vi "DylanScreenTest.vi"() -> ()   [LabVIEW 2019]
uses:
  <userlib>/MicroPython/VIs/uPythonX/uPythonX.xctl
panel:
  in  "Examples":T1(xcontrol)={"VISA Refnum in"="ASRL44::INSTR", "Python Code"="# MicroPython SSD1327 OLED driver examples\n\n# WeMos D1 Mini -- Grove OLED 96x96\n# D1 GPIO5 ------- SCL\n# D2 GPIO4 ------- SDA\n# 3V3 ------------ VCC\n# GND ------------ GND\n\nimport ssd1327\nfrom machine import I2C, Pin\n\n# generic 128x128 SSD1327 OLED\n# i2c = I2C(sda=Pin(4), scl=Pin(5))\n# display = ssd1327.SSD1327_I2C(96, 96, i2c, 60)\n\n# Seeed 96x96 SSD1327 OLED\n#i2c = I2C(sda=Pin(4), scl=Pin(5))\ni2c = I2C(2)\ndisplay = ssd1327.SEEED_OLED_96X96(i2c)\n\n\n# hello world\nfor y in range(0,12):\n     display.text('Hello World', 0, y * 8, 15 - y)\ndisplay.show()\n\n\n# 15 shades of grey\ndisplay.fill(0)\nfor r in range(0,16):\n     display.framebuf.fill_rect(0,r*6,96,6,r)\ndisplay.show()\n\n\n# some text\ndisplay.fill(0)\ndisplay.text('Seeed Studio',0,0,15)\ndisplay.text('Grove OLED',0,10,5)\ndisplay.text('SSD1327',0,20,15)\ndisplay.text('96x96 with',0,30,5)\ndisplay.text('15 shades of',0,40,15)\ndisplay.text('grey using',0,50,5)\ndisplay.text('GS4_HMSB',0,60,15)\ndisplay.text('MicroPython',0,70,5)\ndisplay.text('v1.9 ESP8266',0,80,15)\ndisplay.show()\n\n\n# rotate 180 degrees\ndisplay.rotate(True)\n\n# rotate 0 degrees\ndisplay.write_cmd(0xA2)\ndisplay.write_cmd(0x20)\ndisplay.write_cmd(0xA0)\ndisplay.write_cmd(0x51)\ndisplay.show()\n\n# rotate 0 degrees (flip horizontal)\ndisplay.write_cmd(0xA2)\ndisplay.write_cmd(0x20)\ndisplay.write_cmd(0xA0)\ndisplay.write_cmd(0x52)\ndisplay.show()\n\n# rotate 180 degrees\ndisplay.write_cmd(0xA2)\ndisplay.write_cmd(0x60)\ndisplay.write_cmd(0xA0)\ndisplay.write_cmd(0x42)\ndisplay.show()\n\n# rotate 180 degrees (flip horizontal)\ndisplay.write_cmd(0xA2)\ndisplay.write_cmd(0x60)\ndisplay.write_cmd(0xA0)\ndisplay.write_cmd(0x41)\ndisplay.show()\n\n# rotate 0 degrees\ndisplay.rotate(False)\n\n\n# scroll the framebuf down 16px\ndisplay.fill(0)\ndisplay.text('Hello World', 0, 0, 15)\ndisplay.show()\ndisplay.scroll(0,16)\n\n\n# corner pixels\ndisplay.fill(0)\ndisplay.pixel(0,0,15)\ndisplay.pixel(0,95,15)\ndisplay.pixel(95,95,15)\ndisplay.pixel(95,0,15)\ndisplay.show()\n\n\n# random pixels (slow)\nimport uos\nfor i in range(0,256):\n     x = uos.urandom(1)[0] // 2\n     y = uos.urandom(1)[0] // 2\n     display.pixel(x,y,15)\n     display.show()\n\n\n# invert greyscale lookup table\ndisplay.invert(True)\ndisplay.invert(False)\n\n\n# greyscale lookup\ndisplay.fill(0)\nfor r in range(0,16):\n     display.framebuf.fill_rect(0,r*6,96,6,r)\ndisplay.show()\n\n# more dark shades\ndisplay.lookup([0,2,3,4,5,6,7,8,10,13,16,19,22,25,28])\n\n# more light shades\ndisplay.lookup([0,2,5,8,11,14,16,19,22,23,24,25,26,27,28])\n\n# steps\ndisplay.lookup([0,2,3,6,7,10,11,14,15,19,20,23,24,27,28])\n\n# even more dark shades\ndisplay.lookup([0,2,3,4,5,6,7,8,9,10,11,12,13,20,28])\n\n# revert to default linear scale\ndisplay.write_cmd(0xB9)\n\n\n# greyscale ascii\ndisplay.fill(0)\nfor i in range(32,128):\n     j = (i - 32)\n     x = (j % 12) << 3\n     y = (j // 12) << 3\n     display.text(chr(i), x, y, 1 + (i % 15))\ndisplay.show()\n\n\n# diagonal line pixel by pixel\ndisplay.fill(0)\nfor i in range(0,96):\n     display.pixel(i, i, 15)\n     display.pixel(96 - i, i, 15)\ndisplay.show()\n\n\n# lines using framebuf\ndisplay.fill(0)\nx1 = 0\ny1 = 0\ny2 = 95\nfor x2 in range(0,97,6):\n     display.framebuf.line(x1, y1, x2, y2, 15)\n     display.show()\nx2 = 95\nfor y2 in range(0,97,6):\n     display.framebuf.line(x1, y1, x2, y2, 15)\n     display.show()\n\ndisplay.fill(0)\nx1 = 95\ny1 = 0\ny2 = 95\nfor x2 in range(0,97,6):\n     display.framebuf.line(x1, y1, x2, y2, 15)\n     display.show()\nx2 = 0\nfor y2 in range(0,97,6):\n     display.framebuf.line(x1, y1, x2, y2, 15)\n     display.show()\n\ndisplay.fill(0)\nx1 = 0\ny1 = 95\ny2 = 0\nfor x2 in range(0,97,6):\n     display.framebuf.line(x1, y1, x2, y2, 15)\n     display.show()\nx2 = 95\nfor y2 in range(0,97,6):\n     display.framebuf.line(x1, y1, x2, y2, 15)\n     display.show()\n\ndisplay.fill(0)\nx1 = 95\ny1 = 95\ny2 = 0\nfor x2 in range(0,97,6):\n     display.framebuf.line(x1, y1, x2, y2, 15)\n     display.show()\nx2 = 0\nfor y2 in range(0,97,6):\n     display.framebuf.line(x1, y1, x2, y2, 15)\n     display.show()\n\n\n# rects using framebuf\ndisplay.fill(0)\nfor i in range(0,15):\n     display.framebuf.fill_rect(6 * i, 6 * i, 12, 12, i)\n     display.framebuf.rect(90 - (6 * i), 6 * i, 12, 12, i)\ndisplay.show()\n\n\n# draw a bitmap\n# draw 16x15 smiley in horizontal mode\n# .....#####...... 00 00 0F FF FF 00 00 00\n# ...##.....##.... 00 0F F0 00 00 FF 00 00\n# ..#.........#... 00 F0 00 00 00 00 F0 00\n# .#...........#.. 0F 00 00 00 00 00 0F 00\n# .#...........#.. 0F 00 00 00 00 00 0F 00\n# ###############. FF FF FF FF FF FF FF F0\n# #.#..####..##.#. F0 F0 0F FF F0 0F F0 F0\n# #.#.###.#.###.#. F0 F0 FF F0 F0 FF F0 F0\n# #..###...###..#. F0 0F FF 00 0F FF 00 F0\n# #.............#. F0 00 00 00 00 00 00 F0\n# .#........#..#.. 0F 00 00 00 00 F0 0F 00\n# .#....####...#.. 0F 00 00 FF FF 00 0F 00\n# ..#.........#... 00 F0 00 00 00 00 F0 00\n# ...##.....##.... 00 0F F0 00 00 FF 00 00\n# .....#####...... 00 00 0F FF FF 00 00 00\n\ndata = bytearray([\n0x00, 0x00, 0x0F, 0xFF, 0xFF, 0x00, 0x00, 0x00,\n0x00, 0x0F, 0xF0, 0x00, 0x00, 0xFF, 0x00, 0x00,\n0x00, 0xF0, 0x00, 0x00, 0x00, 0x00, 0xF0, 0x00,\n0x0F, 0x00, 0x00, 0x00, 0x00, 0x00, 0x0F, 0x00,\n0x0F, 0x00, 0x00, 0x00, 0x00, 0x00, 0x0F, 0x00,\n0xFF, 0xFF, 0xFF, 0xFF, 0xFF, 0xFF, 0xFF, 0xF0,\n0xF0, 0xF0, 0x0F, 0xFF, 0xF0, 0x0F, 0xF0, 0xF0,\n0xF0, 0xF0, 0xFF, 0xF0, 0xF0, 0xFF, 0xF0, 0xF0,\n0xF0, 0x0F, 0xFF, 0x00, 0x0F, 0xFF, 0x00, 0xF0,\n0xF0, 0x00, 0x00, 0x00, 0x00, 0x00, 0x00, 0xF0,\n0x0F, 0x00, 0x00, 0x00, 0x00, 0xF0, 0x0F, 0x00,\n0x0F, 0x00, 0x00, 0xFF, 0xFF, 0x00, 0x0F, 0x00,\n0x00, 0xF0, 0x00, 0x00, 0x00, 0x00, 0xF0, 0x00,\n0x00, 0x0F, 0xF0, 0x00, 0x00, 0xFF, 0x00, 0x00,\n0x00, 0x00, 0x0F, 0xFF, 0xFF, 0x00, 0x00, 0x00])\n\n# remap so your data buffer wraps at the desired segment/pixel\n# remapping does not modify the existing ram, instead gives you a window to supply new data\ndisplay.write_cmd(0x15) # SET_COL_ADDR\ndisplay.write_cmd(0x08) # 96x96 oled start pos = 8\ndisplay.write_cmd(0x0F) # start pos + half bitmap width (each byte is 2px wide) = 15\ndisplay.write_cmd(0x75) # SET_ROW_ADDR\ndisplay.write_cmd(0x00) # 96x96 oled start pos = 0\ndisplay.write_cmd(0x1F) # start + bitmap height = 15\ndisplay.write_data(data)\n\ndef bitmap(data,x,y,w,h):\n     display.write_cmd(0x15) # SET_COL_ADDR\n     display.write_cmd(0x08 + (x // 2))\n     display.write_cmd(0x08 + (x // 2) + (w // 2))\n     display.write_cmd(0x75) # SET_ROW_ADDR\n     display.write_cmd(0x00 + y)\n     display.write_cmd(y + h)\n     display.write_data(data)\n\n\nfor y in range(0,6):\n     for x in range(0,6):\n          bitmap(data, x * 16, y * 16, 15, 15)"}
  in  "ssd1327":T1(xcontrol)={"VISA Refnum in"="ASRL44::INSTR", "Python Code"="'''\nMicroPython SSD1327 OLED I2C driver\nhttps://github.com/mcauser/micropython-ssd1327\nMIT License\nCopyright (c) 2017 Mike Causer\nPermission is hereby granted, free of charge, to any person obtaining a copy\nof this software and associated documentation files (the \"Software\"), to deal\nin the Software without restriction, including without limitation the rights\nto use, copy, modify, merge, publish, distribute, sublicense, and/or sell\ncopies of the Software, and to permit persons to whom the Software is\nfurnished to do so, subject to the following conditions:\nThe above copyright notice and this permission notice shall be included in all\ncopies or substantial portions of the Software.\nTHE SOFTWARE IS PROVIDED \"AS IS\", WITHOUT WARRANTY OF ANY KIND, EXPRESS OR\nIMPLIED, INCLUDING BUT NOT LIMITED TO THE WARRANTIES OF MERCHANTABILITY,\nFITNESS FOR A PARTICULAR PURPOSE AND NONINFRINGEMENT. IN NO EVENT SHALL THE\nAUTHORS OR COPYRIGHT HOLDERS BE LIABLE FOR ANY CLAIM, DAMAGES OR OTHER\nLIABILITY, WHETHER IN AN ACTION OF CONTRACT, TORT OR OTHERWISE, ARISING FROM,\nOUT OF OR IN CONNECTION WITH THE SOFTWARE OR THE USE OR OTHER DEALINGS IN THE\nSOFTWARE.\n'''\n\nfrom micropython import const\nimport time\nimport framebuf\n\n\n# commands\nSET_COL_ADDR          = const(0x15)\nSET_SCROLL_DEACTIVATE = const(0x2E)\nSET_ROW_ADDR          = const(0x75)\nSET_CONTRAST          = const(0x81)\nSET_SEG_REMAP         = const(0xA0)\nSET_DISP_START_LINE   = const(0xA1)\nSET_DISP_OFFSET       = const(0xA2)\nSET_DISP_MODE         = const(0xA4) # 0xA4 normal, 0xA5 all on, 0xA6 all off, 0xA7 when inverted\nSET_MUX_RATIO         = const(0xA8)\nSET_FN_SELECT_A       = const(0xAB)\nSET_DISP              = const(0xAE) # 0xAE power off, 0xAF power on\nSET_PHASE_LEN         = const(0xB1)\nSET_DISP_CLK_DIV      = const(0xB3)\nSET_SECOND_PRECHARGE  = const(0xB6)\nSET_GRAYSCALE_TABLE   = const(0xB8)\nSET_GRAYSCALE_LINEAR  = const(0xB9)\nSET_PRECHARGE         = const(0xBC)\nSET_VCOM_DESEL        = const(0xBE)\nSET_FN_SELECT_B       = const(0xD5)\nSET_COMMAND_LOCK      = const(0xFD)\n\n# registers\nREG_CMD  = const(0x80)\nREG_DATA = const(0x40)\n\n\nclass SSD1327:\n     def __init__(self, width, height, external_vcc):\n          self.width = width\n          self.height = height\n          self.external_vcc = external_vcc\n          self.buffer = bytearray(self.width * self.height // 2)\n          self.framebuf = framebuf.FrameBuffer(self.buffer, self.width, self.height, framebuf.GS4_HMSB)\n          self.poweron()\n          self.init_display()\n\n     def init_display(self):\n          for cmd in (\n               SET_COMMAND_LOCK, 0x12, # Unlock\n               SET_DISP, # Display off\n               # Resolution and layout\n               SET_DISP_START_LINE, 0x00,\n               SET_DISP_OFFSET, 0x20, # Set vertical offset by COM from 0~127\n               # Set re-map\n               # Enable column address re-map\n               # Disable nibble re-map\n               # Horizontal address increment\n               # Enable COM re-map\n               # Enable COM split odd even\n               SET_SEG_REMAP, 0x51,\n               SET_MUX_RATIO, self.height - 1,\n               # Timing and driving scheme\n               SET_FN_SELECT_A, 0x01, # Enable internal VDD regulator\n               SET_PHASE_LEN, 0x51, # Phase 1: 1 DCLK, Phase 2: 5 DCLKs\n               SET_DISP_CLK_DIV, 0x01, # Divide ratio: 1, Oscillator Frequency: 0\n               SET_PRECHARGE, 0x08, # Set pre-charge voltage level: VCOMH\n               SET_VCOM_DESEL, 0x07, # Set VCOMH COM deselect voltage level: 0.86*Vcc\n               SET_SECOND_PRECHARGE, 0x01, # Second Pre-charge period: 1 DCLK\n               SET_FN_SELECT_B, 0x62, # Enable enternal VSL, Enable second precharge\n               # Display\n               SET_GRAYSCALE_LINEAR, # Use linear greyscale lookup table\n               SET_CONTRAST, 0x7f, # Medium brightness\n               SET_DISP_MODE, # Normal, not inverted\n               # 96x96:\n               # SET_ROW_ADDR, 0 95,\n               # SET_COL_ADDR, 8, 55,\n               # 128x128:\n               # SET_ROW_ADDR, 0 127,\n               # SET_COL_ADDR, 0, 63,\n               SET_ROW_ADDR, 0x00, self.height - 1,\n               SET_COL_ADDR, ((128 - self.width) // 4), 63 - ((128 - self.width) // 4),\n\n               SET_SCROLL_DEACTIVATE,\n               SET_DISP | 0x01): # Display on\n               self.write_cmd(cmd)\n          self.fill(0)\n          self.show()\n\n     def poweroff(self):\n          self.write_cmd(SET_FN_SELECT_A)\n          self.write_cmd(0x00) # Disable internal VDD regulator, to save power\n          self.write_cmd(SET_DISP)\n\n     def poweron(self):\n          self.write_cmd(SET_FN_SELECT_A)\n          self.write_cmd(0x01) # Enable internal VDD regulator\n          self.write_cmd(SET_DISP | 0x01)\n\n     def contrast(self, contrast):\n          self.write_cmd(SET_CONTRAST)\n          self.write_cmd(contrast) # 0-255\n\n     def invert(self, invert):\n          self.write_cmd(SET_DISP_MODE | (invert & 1) << 1 | (invert & 1)) # 0xA4=Normal, 0xA7=Inverted\n\n     def show(self):\n          self.write_cmd(SET_COL_ADDR)\n          self.write_cmd((128 - self.width) // 4)\n          self.write_cmd(63 - ((128 - self.width) // 4))\n          self.write_cmd(SET_ROW_ADDR)\n          self.write_cmd(0x00)\n          self.write_cmd(self.height - 1)\n          self.write_data(self.buffer)\n\n     def fill(self, col):\n          self.framebuf.fill(col)\n\n     def pixel(self, x, y, col):\n          self.framebuf.pixel(x, y, col)\n\n     def scroll(self, dx, dy):\n          self.framebuf.scroll(dx, dy)\n          # software scroll\n\n     def text(self, string, x, y, col=15):\n          self.framebuf.text(string, x, y, col)\n\n\nclass SSD1327_I2C(SSD1327):\n     def __init__(self, width, height, i2c, addr=0x3c, external_vcc=False):\n          self.i2c = i2c\n          self.addr = addr\n          self.temp = bytearray(2)\n          super().__init__(width, height, external_vcc)\n\n     def write_cmd(self, cmd):\n          self.temp[0] = REG_CMD # Co=1, D/C#=0\n          self.temp[1] = cmd\n          self.i2c.writeto(self.addr,self.temp)\n\n     def write_data(self, buf):\n          self.i2c.writeto(self.addr,b'@' + buf)\n\nclass SEEED_OLED_96X96(SSD1327_I2C):\n     def __init__(self, i2c):\n          super().__init__(96, 96, i2c)\n\n     def rotate(self, rotate):\n          self.poweroff()\n          self.write_cmd(SET_DISP_OFFSET)\n          self.write_cmd(0x60 if rotate else 0x20) # 0x20=0 degrees, 0x60=180 degrees\n          self.write_cmd(SET_SEG_REMAP)\n          self.write_cmd(0x42 if rotate else 0x51) # 0x51=0 degrees, 0x42=180 degrees\n          self.poweron()\n\n     def lookup(self, table):\n          # GS0 has no pre-charge and current drive\n          self.write_cmd(SET_GRAYSCALE_TABLE)\n          for i in range(0,15):\n               self.write_cmd(table[i])\n"}
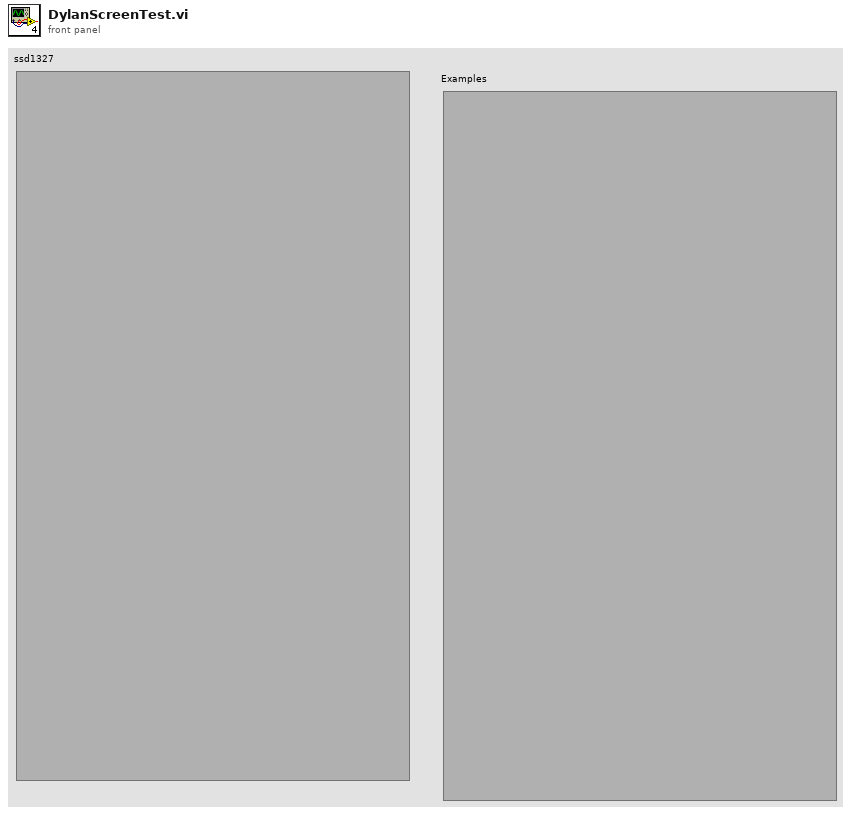
[diagram p1: front panel]
types:
  T1 = cluster{"VISA Refnum in":refnum<visa-resource-name>, "Python Code":string}
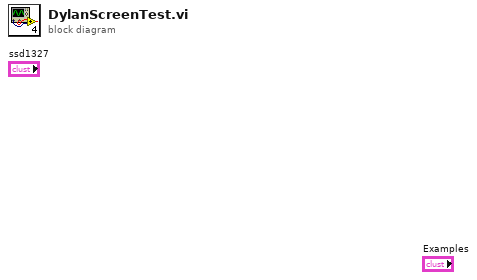
[diagram p0: block diagram]
diagram:
